vi "Large File - Generate report graphs.vi"(8 "error in (no error)":errorcluster, 9 "Test Energies":dbl[](array[numeric]), 10 "report file path":path, 11 "file path":path) -> (0 "error out":errorcluster)   [LabVIEW 2015]
uses:
  <vilib>/addons/_office/word.llb/Word Easy Table (num).vi
  <vilib>/Utility/NIReport.llb/NI_report.lvclass
  <vilib>/Utility/NIReport.llb/Word/NI_Word.lvclass
  <vilib>/addons/_office/NI_ReportGenerationToolkit.lvlib
panel:
  out "Min and Max Temperatures":dbl[][](array[numeric])
  out "Full Shot - Discharge Voltage (V) and Current (A) against Time (s)":waveform(dbl)[](graph)
  out "Temperature (Degrees C) against Time (s)":waveform(dbl)(graph)
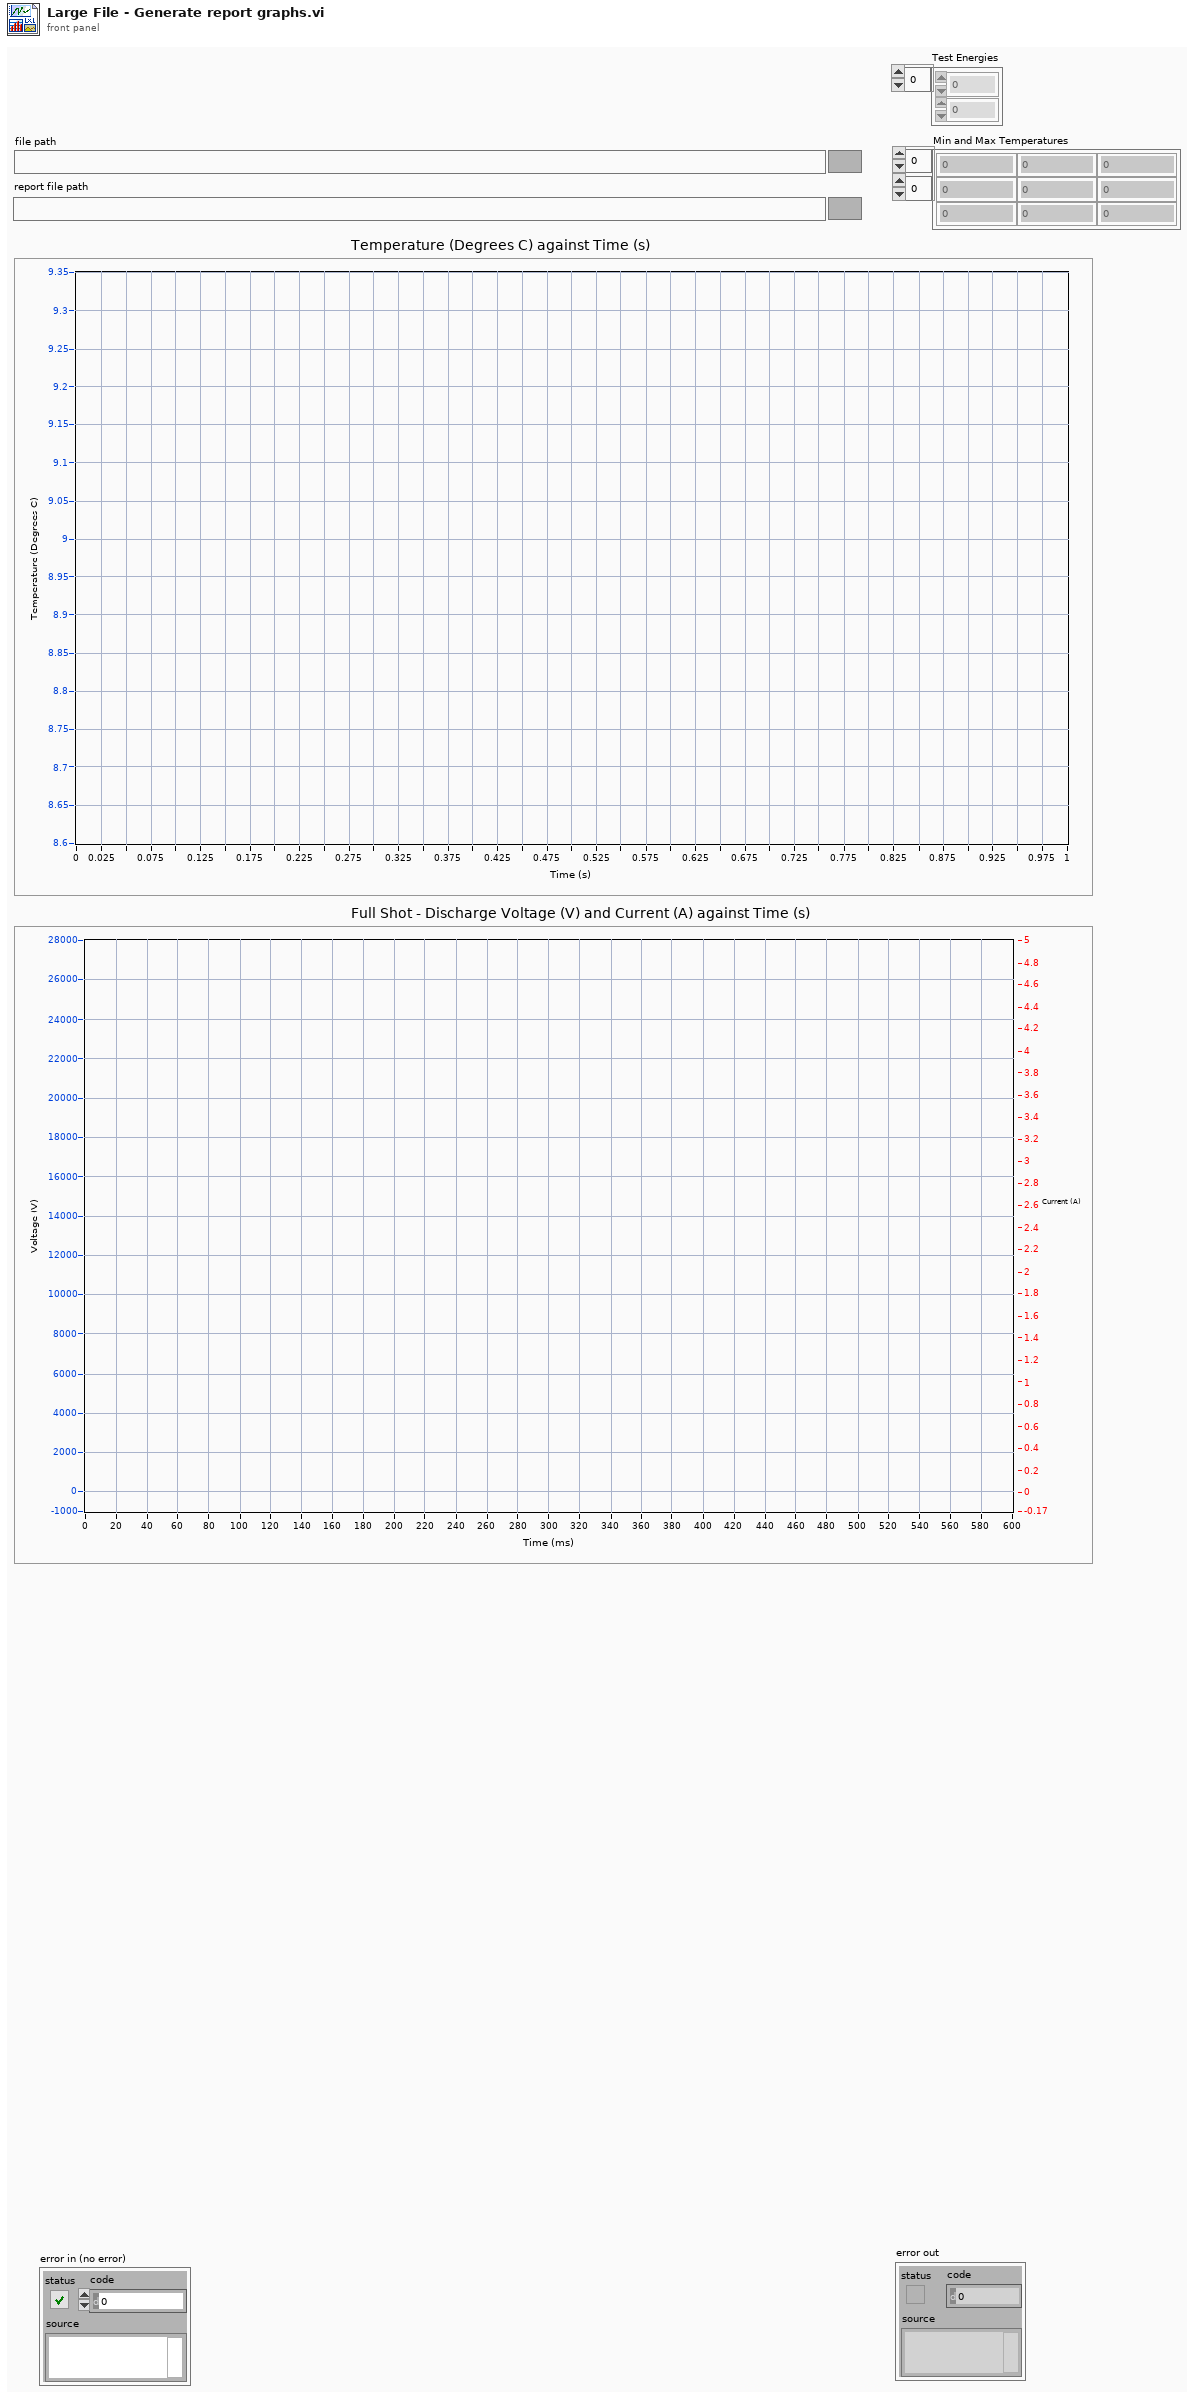
[diagram p1: front panel]
types:
  T1 = enum16{"Standard Report", "HTML", "Word", "Excel"}
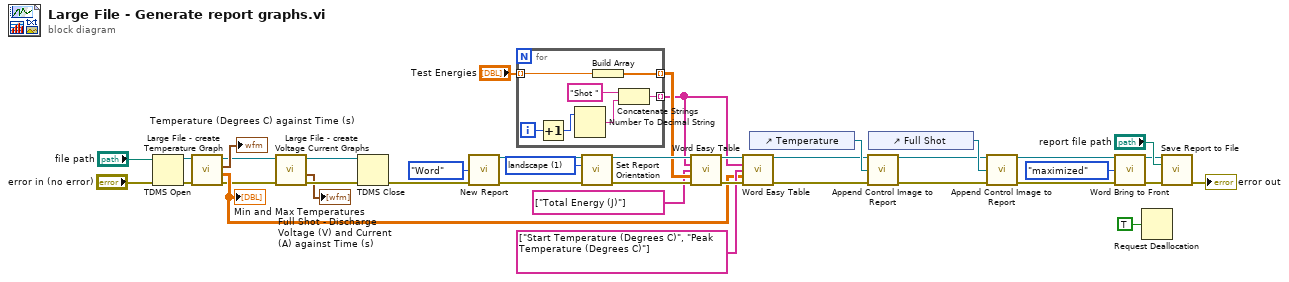
[diagram p0: block diagram]
diagram:
  w35 = 1 items=["portrait", "landscape"] ("orientation (portrait)")
  n1 = TDMS Open(8:"error in (no error)", 11:"file path") -> (0:w10:errorcluster, 3:w11:refnum<k34>)  [unwired: 5 in]
  n2 = call "Large File - create Temperature Graph.vi"("error in (no error)"=w10, "tdms file"=w11) -> ("error out"=w6:errorcluster, "Min and Max Temperatures"=w8:dbl[][], "Temperature (Degrees C) against Time (s)"=→"Temperature (Degrees C) against Time (s)":waveform(dbl), "tdms file out"=w7:refnum<k34>)  [unwired: 2 in]
  "Min and Max Temperatures" <- w8
  n3 = call "Large File - create Voltage Current Graphs.vi"("error in (no error)"=w6, "tdms file"=w7) -> ("error out"=w4:errorcluster, "Single Shot - Discharge Voltage (V) and Current (A) against Time (s)"=→"Full Shot - Discharge Voltage (V) and Current (A) against Time (s)":waveform(dbl)[], "tdms file out"=w5:refnum<k34>)  [unwired: 2 in, 1 out]
  n4 = TDMS Close(8:w4, 11:w5) -> (0:w33:errorcluster)  [unwired: 1 out]
  n5 = call <vilib>:"New Report.vi"("report type"=T1."Word", "error in (no error)"=w33) -> ("report out"=w37:refnum<class "NI_report.lvclass">, "error out"=w36:errorcluster)  [unwired: 12 in]
  n6 = for {
    tunnel: "Test Energies" -> [w43] mode=indexing
    tunnel: [w44] -> w14 mode=indexing
    tunnel: [w42] -> w20 mode=indexing
    i -> [w41]
    n7 = Increment(x=w41) -> (x+1=w40:i32)
    n8 = Number To Decimal String(number=w40) -> (decimal integer string=w45:string)  [unwired: 1 in]
    n9 = Build Array(w43) -> (w42:dbl[])
    n10 = Concatenate Strings("Shot ", w45) -> (w44:string)
  }
  n11 = call-dynamic "Set Report Orientation.vi"("report in"=w37, "orientation (portrait)"=w35, "error in (no error)"=w36) -> ("report out"=w22:refnum<class "NI_report.lvclass">, "error out"=w23:errorcluster)  [unwired: 11 in]
  n12 = call-poly <vilib>:"Word Easy Table.vi"("report in"=w22, "row headers"=w14, "column headers"=string[] ["Total Energy (J)"], "text data"=w20, "error in (no error)"=w23) -> ("report out"=w15:refnum<class "NI_report.lvclass">, "error out"=w16:errorcluster)  [unwired: 8 in, 1 out]
  n13 = call-poly <vilib>:"Word Easy Table.vi"("report in"=w15, "row headers"=w14, "column headers"=string[] ["Start Temperature (Degrees C)", "Peak Temperature (Degrees C)"], "text data"=w8, "error in (no error)"=w16) -> ("report out"=w18:refnum<class "NI_report.lvclass">, "error out"=w17:errorcluster)  [unwired: 8 in, 1 out]
  n14 = control-ref of="Temperature"() -> (w32:refnum<vi>)
  n15 = call-dynamic "Append Control Image to Report.vi"("report in"=w18, "ctrl reference"=w32, "error in (no error)"=w17) -> ("report out"=w2:refnum<class "NI_report.lvclass">, "error out"=w1:errorcluster)  [unwired: 9 in, 2 out]
  n16 = control-ref of="Full Shot"() -> (w31:refnum<vi>)
  n17 = call-dynamic "Append Control Image to Report.vi"("report in"=w2, "ctrl reference"=w31, "error in (no error)"=w1) -> ("report out"=w28:refnum<class "NI_report.lvclass">, "error out"=w27:errorcluster)  [unwired: 9 in, 2 out]
  n18 = call <vilib>:"Word Bring to Front.vi"("report in"=w28, "window state (maximized)"=enum16{"maximized", "minimized", "normal"}."maximized", "error in (no error)"=w27) -> ("report out"=w30:refnum<class "NI_report.lvclass">, "error out"=w29:errorcluster)  [unwired: 11 in]
  n19 = Request Deallocation(TRUE ("flag")) -> ()
  n20 = call-dynamic "Save Report to File.vi"("report in"=w30, "report file path"="report file path", "error in (no error)"=w29) -> ("error out"=→"error out":errorcluster)  [unwired: 11 in, 1 out]
